vi "Get Events.vi"(11 "Loading Dialog View in":refnum<class "Loading Dialog View.lvclass">) -> (2 "Events":T1, 3 "Loading Dialog View out":refnum<class "Loading Dialog View.lvclass">)   [LabVIEW 2013, in "Loading Dialog View.lvlib" / "Loading Dialog View.lvclass"]
uses:
  Loading Dialog View.lvclass
  Typedef/Events.ctl
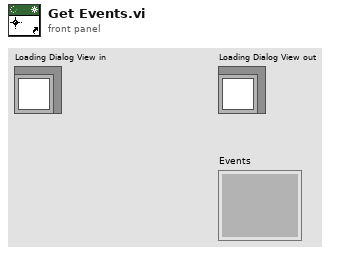
[diagram p1: front panel]
types:
  T1 = typedef "Loading Dialog View.lvlib/Loading Dialog View.lvclass/Events.ctl" = cluster{}
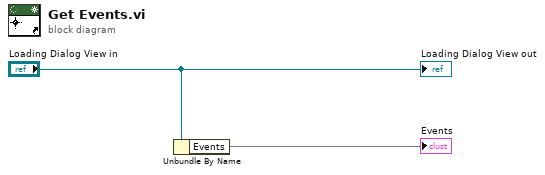
[diagram p0: block diagram]
diagram:
  n1 = Unbundle By Name("Loading Dialog View in") -> ("Events"=→"Events")
  "Loading Dialog View out" <- "Loading Dialog View in"
